vi "Get SMO HELP.vi"(8 "error in (no error)":errorcluster, 10 "Command":string, 11 "Instrument.Framework-Template in":refnum<class "Instrument.Framework-Template.lvclass">) -> (0 "error out":errorcluster, 2 "output cluster":T1, 3 "Instrument.Framework-Template out":refnum<class "Instrument.Framework-Template.lvclass">)   [LabVIEW 2019, in "Instrument.Framework-Template.lvclass"]
uses:
  Instrument.Framework-Template.lvclass
  <userlib>/LevyLab/Instrument Framework/subsystems/Help/typedefs/Help--cluster.ctl
  Typedefs/Instrument.Framework-Template.PublicCommands--Enum.ctl
  <userlib>/LevyLab/Instrument Framework/Instrument Types/SCPI/Instrument.SCPI.lvclass
  <userlib>/LevyLab/Instrument Framework/subsystems/Help/Help.lvclass
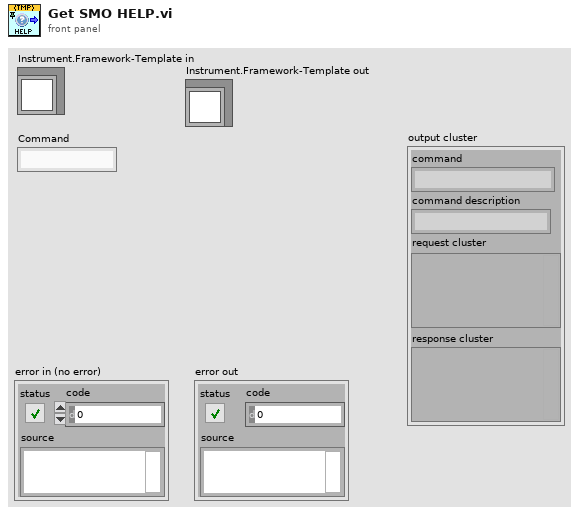
[diagram p1: front panel]
types:
  T1 = typedef "Instrument.lvlib/Help.lvclass/Help--cluster.ctl" = cluster{"command":string, "command description":string, "request cluster":variant, "response cluster":variant}
  T2 = typedef "Instrument.Framework-Template.lvclass/Instrument.Framework-Template.PublicCommands--Enum.ctl" = enum16{"doSomething"}
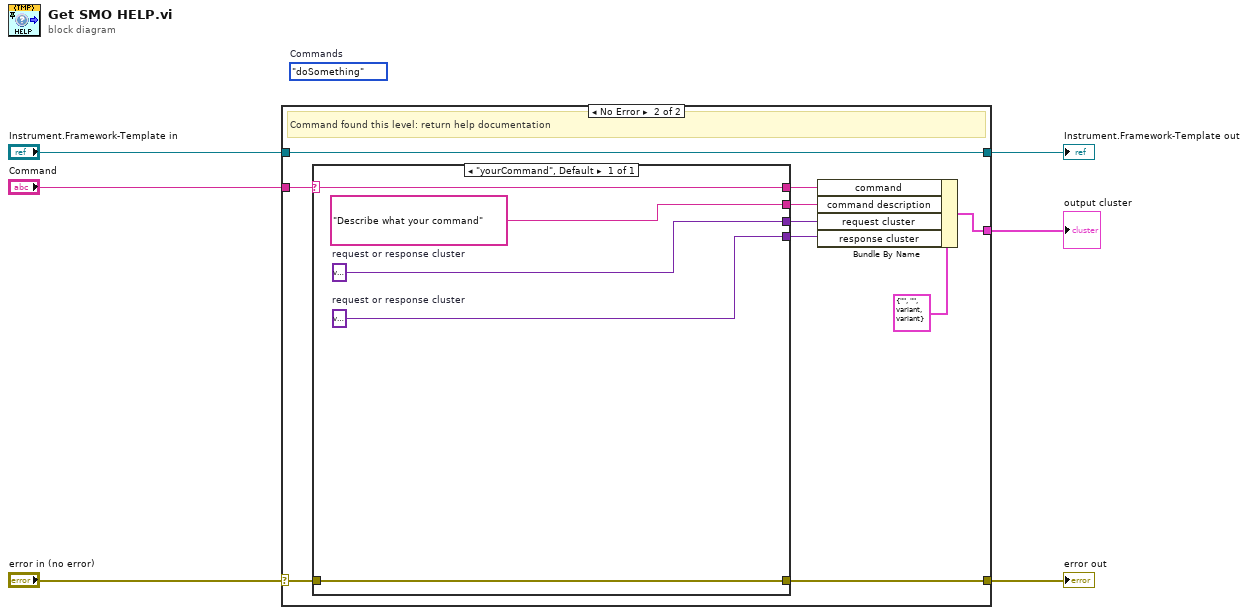
[diagram p0: block diagram]
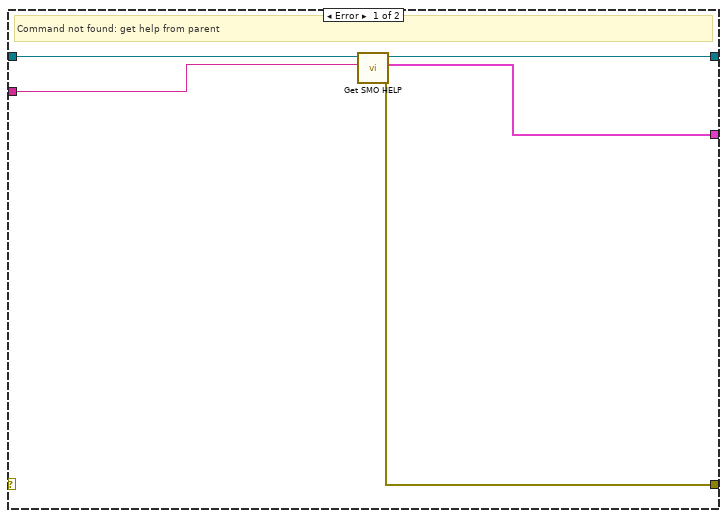
[diagram p2: hidden frame]
diagram:
  (unwired) Instrument.Framework-Template.PublicCommands--Enum."doSomething"  # Commands
  n1 = case shown="No Error" "error in (no error)" {
    selector: "error in (no error)" -> [_ w16]
    tunnel: "Instrument.Framework-Template in" -> [w11 w21]
    tunnel: [w10 w21] -> w5
    tunnel: [w8 w15] -> w6
    tunnel: [w7 w20] -> w4
    tunnel: "Command" -> [w9 w18]
    frame Error {
      # "Command not found: get help from parent"
      n2 = call-parent "Get SMO HELP.vi"("Command"=w9, "Instrument in"=w11) -> ("error out"=w8:errorcluster, "help cluster"=w7:T1, "Instrument out"=w10:refnum<class "Instrument.Framework-Template.lvclass">)  [unwired: 7 in]
    }
    frame No Error {
      # "Command found this level: return help documentation"
      n3 = case shown="\"yourCommand\", Default" w18 {
        selector: w18 -> [w26]
        tunnel: [w26] -> w17
        tunnel: w16 -> [w25]
        tunnel: [w25] -> w15
        tunnel: ["Describe what your command"] -> w14
        tunnel: [w23] -> w13
        tunnel: [w22] -> w12
        frame "yourCommand", Default {
          w23 = variant  # request or response cluster
          w22 = variant  # request or response cluster
        }
      }
      n4 = Bundle By Name(cluster=T1 {"command"="", "command description"="", "request cluster"=variant, "response cluster"=variant} ("Help"), "command"=w17, "command description"=w14, "request cluster"=w13, "response cluster"=w12) -> (w20:T1)
    }
  }
  "Instrument.Framework-Template out" <- w5
  "output cluster" <- w4
  "error out" <- w6
